vi "STDBGA_获取温度和叶绿素值.vi"(8 "error in (no error)":errorcluster caption="错误输入（无错误）", 11 "MB session in":refnum<class "MB_Master.lvclass">) -> (0 "error out":errorcluster caption="错误输出", 2 "STD藻密度":cluster{"温度测量值":sgl, "测试值":dbl, "信号值":sgl}, 3 "MB session out":refnum<class "MB_Master.lvclass">)   [LabVIEW 2022 SP3, in "斯坦道多参数.lvlib"]
uses:
  <vilib>/Plasmionique/MB Master/MB_Master/MB_Master.lvclass
  <vilib>/Plasmionique/MB Master/MB Master.lvlib
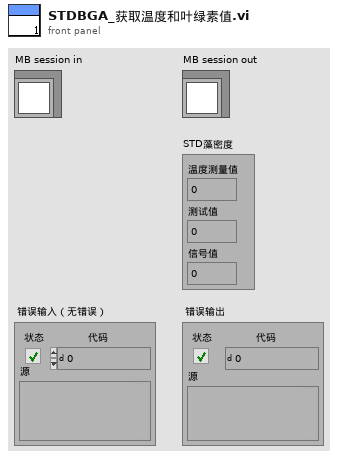
[diagram p1: front panel]
types:
  T1 = cluster{"pH":u32, "DO":u32, "Cond":u32, "Turb":u32, "叶绿素a":u32, "藻密度":u32, "ORP":u32, "COD":u32, "氯化物":u32, "氨氮":u32, "水中油":u32, "悬浮物":u32, "余氯":u32}
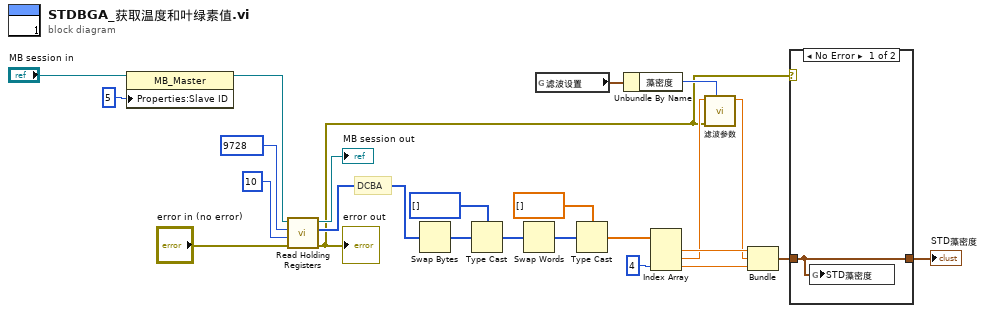
[diagram p0: block diagram]
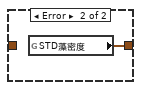
[diagram p2: hidden frame]
diagram:
  # "DCBA"
  n1 = property class="MB_Master"(reference="MB session in", "Properties:Slave ID"=u16 5 ("y")) -> (reference out=w15:refnum<class "MB_Master.lvclass">)  [unwired: 1 in, 1 out]
  n2 = call <vilib>:"Read Holding Registers.vi"("error in (no error)"="error in (no error)", "quantity"=u16 10, "starting address"=u16 9728, "MB session in"=w15) -> ("error out"=w5:errorcluster, "Registers"=w13:u16[], "MB session out"=→"MB session out":refnum<class "MB_Master.lvclass">)  [unwired: 5 in]
  "error out" <- w5
  n3 = Swap Bytes(anything=w13) -> (byte swapped=w2:u16[])
  n4 = Type Cast(type=u32[] [] ("数组 2"), x=w2) -> (*(type *) &x=w20:u32[])
  n5 = Swap Words(1:w20) -> (0:w22:u32[])
  n6 = global read "断电保存变量.vi" "滤波设置"() -> (w7:T1)
  n7 = Type Cast(type=sgl[] [] ("数组 2"), x=w22) -> (*(type *) &x=w18:sgl[])
  n8 = Unbundle By Name(w7) -> ("藻密度"=w6:u32)
  n9 = Index Array(array=w18, index #3=4 ("索引")) -> (element #1=w17:sgl, element #2=w9:sgl, element #3=w3:sgl)  [unwired: 2 in]
  n10 = call "滤波参数.vi"("滤波次数"=w6, "error in (no error)"=w5, "x"=w9) -> ("mode"=w8:dbl)  [unwired: 7 in, 1 out]
  n11 = Bundle("数值"=w17, "mode"=w8, "数值"=w3) -> (w12:cluster{"数值":sgl, "mode":dbl, "数值":sgl})  [unwired: 1 in]
  n12 = case shown="No Error" w5 {
    tunnel: w12 -> [w25 _]
    tunnel: [w25 w26] -> w1
    frame No Error {
      n13 = global write "禹山过程全局变量.vi" "STD藻密度"(w25) -> ()
    }
    frame Error {
      n14 = global read "禹山过程全局变量.vi" "STD藻密度"() -> (w26:cluster{"温度测量值":sgl, "测量值":sgl, "信号值":sgl})
    }
  }
  "STD藻密度" <- w1
